vi "Create DSFPluginSettings.vi"(8 "error in (no error)":errorcluster, 9 "user settings":variant, 10 "id":string, 11 "DSFPluginSettings in":refnum<class "DSFPluginSettings.lvclass">) -> (0 "error out":errorcluster, 3 "DSFPluginSettings out":refnum<class "DSFPluginSettings.lvclass">)   [LabVIEW 2017, in "DSFPluginSettings.lvclass"]
uses:
  DSFPluginSettings.lvclass
  DSFPluginSettings.lvclass/DSFPluginSettings.ctl
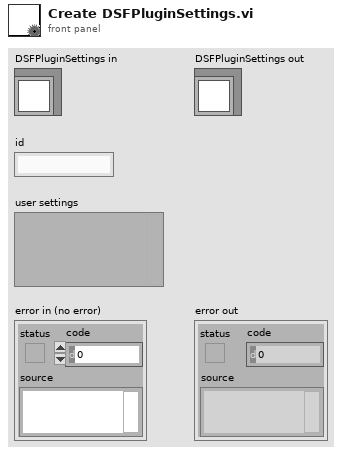
[diagram p1: front panel]
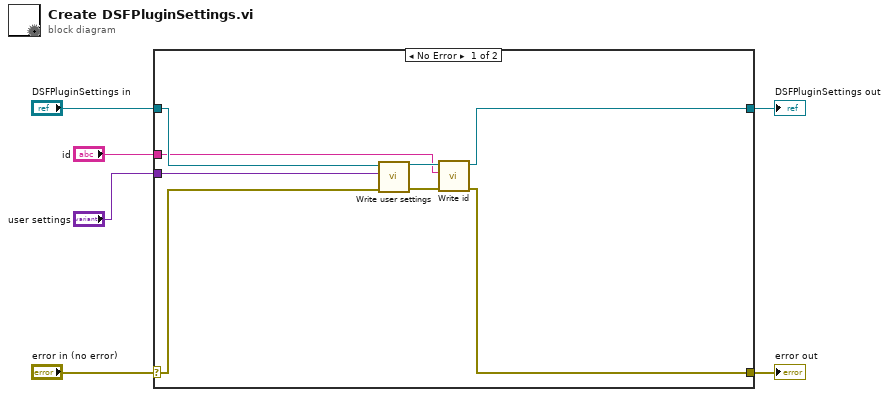
[diagram p0: block diagram]
diagram:
  n1 = case shown="No Error" "error in (no error)" {
    selector: "error in (no error)" -> [w9 w16]
    tunnel: [w10 w16] -> w5
    tunnel: [w11 w15] -> w3
    tunnel: "DSFPluginSettings in" -> [w14 w15]
    tunnel: "id" -> [w8 _]
    tunnel: "user settings" -> [w7 _]
    frame No Error {
      n2 = call "Write user settings.vi"("error in (no error)"=w9, "user settings"=w7, "DSFPluginSettings in"=w14) -> ("error out"=w12:errorcluster, "DSFPluginSettings out"=w13:refnum<class "DSFPluginSettings.lvclass">)  [unwired: 7 in]
      n3 = call "Write id.vi"("error in (no error)"=w12, "id"=w8, "DSFPluginSettings in"=w13) -> ("error out"=w10:errorcluster, "DSFPluginSettings out"=w11:refnum<class "DSFPluginSettings.lvclass">)  [unwired: 7 in]
    }
    frame Error {
    }
  }
  "error out" <- w5
  "DSFPluginSettings out" <- w3
